vi "all vi close.vi"() -> ()   [LabVIEW 2017]
panel:
  out "PLC 5":bool
  out "PLC 2":bool
  out "PLC 4":bool
  out "PLC 3":bool
  out "PLC 1":bool
  in  "ST3_Barcode 21":string
  out "St3E":bool
  out "St2E":bool
  out "St1E":bool
  in  "INTERLOCK_03":u16
  out "ST3_inerlock":bool
  out "ST2_inerlock":bool
  in  "INTERLOCK_02":u16
  out "ST1_inerlock":bool
  in  "INTERLOCK_01":u16
  in  "ST3_Barcode2":string
  in  "ST3_Barcode1":string
  out "ST_3CC":bool
  in  "ST3_Barcode":string
  in  "ST2_Barcode":string
  out "ST_2CC":bool
  in  "ST1_Barcode":string
  out "ST_1CC":bool
  out "all vi close":bool
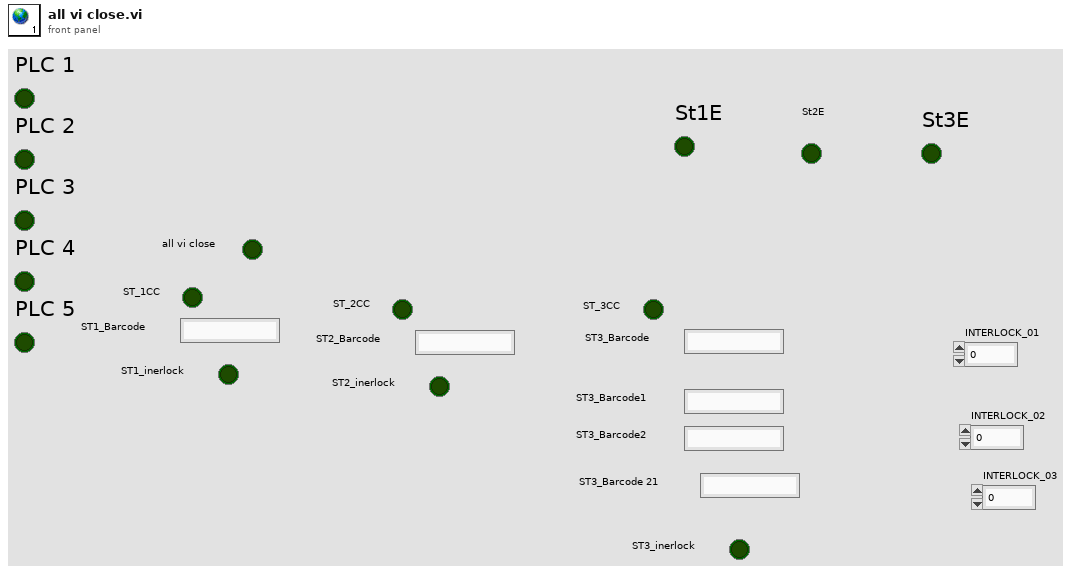
[diagram p1: front panel]
diagram:
